vi "Read Available Measurements.vi"(8 "error in (no error)":errorcluster, 11 "Controller in":refnum<class "Controller.lvclass">) -> (0 "error out":errorcluster, 2 "Available Measurements":string[](array[string]), 3 "Controller out":refnum<class "Controller.lvclass">)   [LabVIEW 2015, in "Controller Actor.lvlib" / "Controller.lvclass"]
uses:
  Controller.lvclass
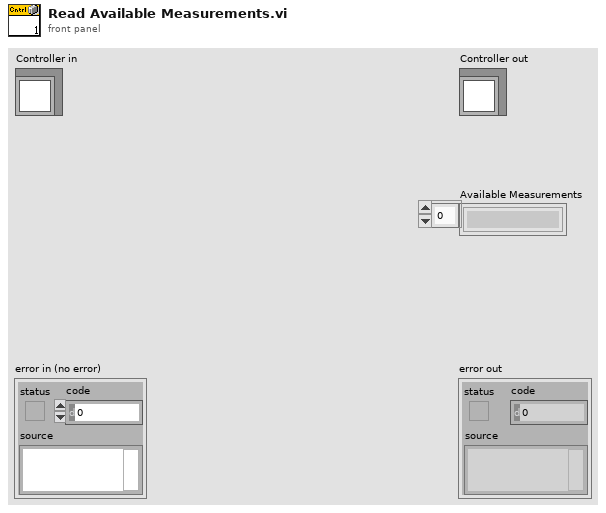
[diagram p1: front panel]
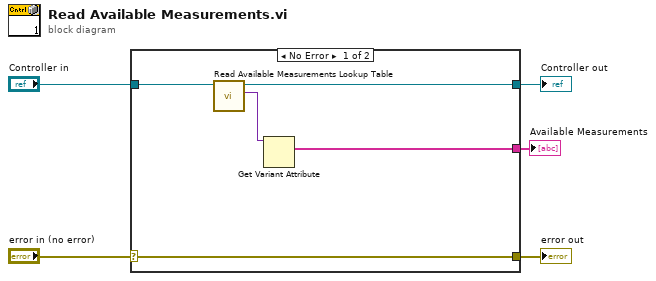
[diagram p0: block diagram]
diagram:
  n1 = case shown="No Error" "error in (no error)" {
    selector: "error in (no error)" -> [w10 w11]
    tunnel: [w10 w11] -> w4
    tunnel: [w6 w12] -> w2
    tunnel: "Controller in" -> [w7 w12]
    tunnel: [w8 _] -> w1
    frame No Error {
      n2 = call "Read Available Measurements Lookup Table.vi"("Controller in"=w7) -> ("Available Measurements Lookup Table"=w9:variant, "Controller out"=w6:refnum<class "Controller.lvclass">)  [unwired: 8 in, 1 out]
      n3 = Get Variant Attribute(Variant=w9) -> (names=w8:string[])  [unwired: 3 in, 3 out]
    }
    frame Error {
    }
  }
  "error out" <- w4
  "Controller out" <- w2
  "Available Measurements" <- w1
